vi "respuesta read adc.vi"(8 "error in (no error)":errorcluster, 11 "Arduino in":refnum<class "Arduino.lvclass">) -> (0 "error out":errorcluster, 2 "salida":string, 3 "Arduino out":refnum<class "Arduino.lvclass">)   [LabVIEW 2019, in "Arduino.lvclass"]
uses:
  Arduino.lvclass
  Arduino.lvclass/Arduino.ctl
  Serial Device.lvclass
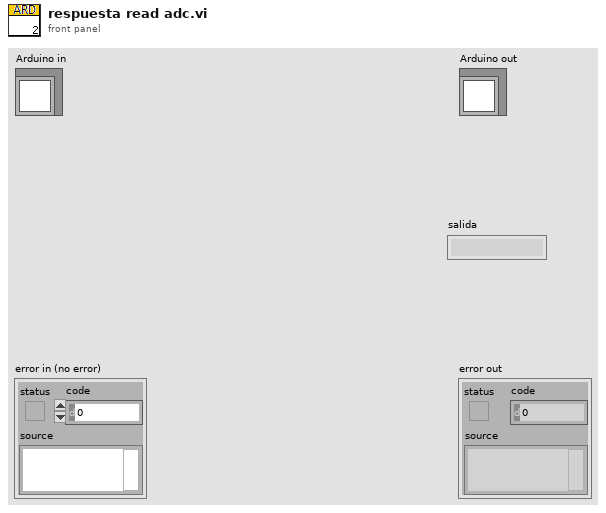
[diagram p1: front panel]
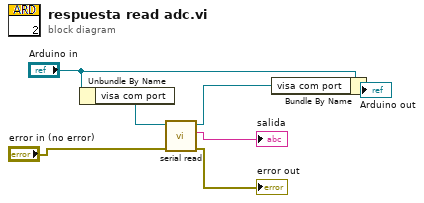
[diagram p0: block diagram]
diagram:
  n1 = Unbundle By Name("Arduino in") -> ("visa com port"=w7:refnum<visa-resource-name>)
  n2 = call "serial read.vi"("error in (no error)"="error in (no error)", "VISA resource name"=w7) -> ("error out"=→"error out":errorcluster, "respuesta serial"=→"salida":string, "VISA resource nameout"=w4:refnum<visa-resource-name>)  [unwired: 7 in]
  n3 = Bundle By Name(cluster="Arduino in", "visa com port"=w4) -> (→"Arduino out":refnum<class "Arduino.lvclass">)
